vi "Test with main menus.vi"() -> ()   [LabVIEW 2019]
uses:
  Menu From Cluster.lvlib
panel:
  out "Item":string
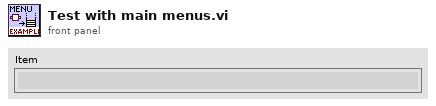
[diagram p1: front panel]
types:
  T1 = cluster{"Sub Enum":enum16{"Item1", "Item2", "Item3"}, "Sub Boolean":bool, "Subsubcluster":cluster{"Sub Enum":enum16{"Item1", "Item2", "Item3"}, "Sub Boolean":bool}}
  T2 = cluster{"An Enum":enum16{"Item1", "Item2", "Item3"}, "A Boolean":bool, "Another boolean":bool}
  T3 = cluster{"Options Menu":cluster{"An Enum":enum16{"Item1", "Item2", "Item3"}, "A Boolean":bool, "Another boolean":bool}}
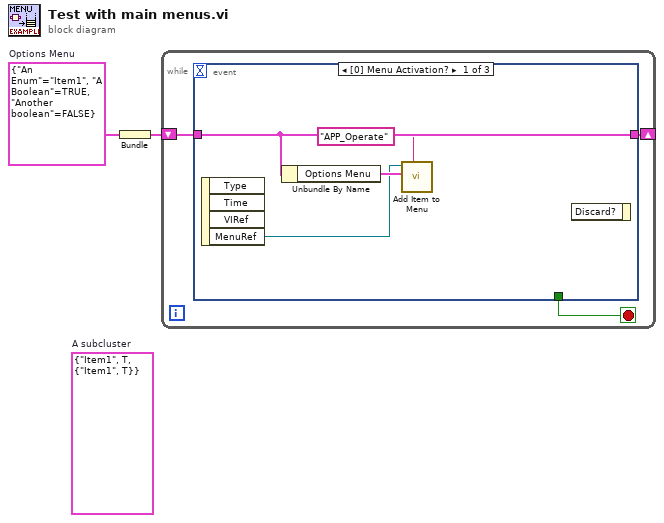
[diagram p0: block diagram]
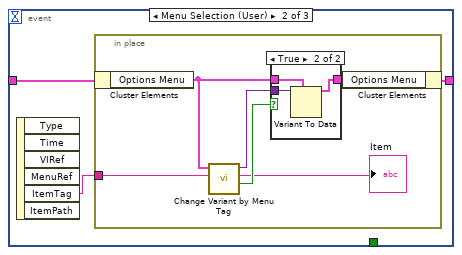
[diagram p2: hidden frame]
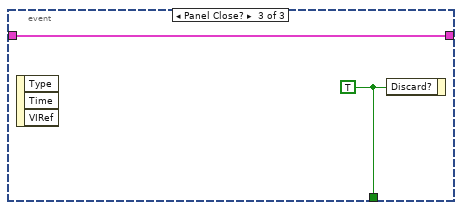
[diagram p4: hidden frame]
diagram:
  (unwired) T1 {"Sub Enum"=enum."Item1", "Sub Boolean"=TRUE, "Subsubcluster"={"Sub Enum"=enum."Item1", "Sub Boolean"=TRUE}}  # A subcluster
  w1 = T2 {"An Enum"=enum."Item1", "A Boolean"=TRUE, "Another boolean"=FALSE}  # Options Menu
  n1 = Bundle("Options Menu"=w1) -> (w2:T3)  [unwired: 1 in]
  n2 = while {
    shift-right: [w4] -> _
    shift-left: w2 -> [w5]
    stop <- w3 stop-if-true
    n3 = event shown="[0] Menu Activation?" {
      selector: _ -> [_ _ _]
      dyn-events: _ -> [_ _ _]
      timeout: _ -> [_ _ _]
      tunnel: w5 -> [w9 w12 w24]
      tunnel: [w9 w11 w24] -> w4
      tunnel: [_ _ w23] -> w3
      event Menu Activation? {
        n4 = event-data() -> ("MenuRef"=w7:refnum<k9>)  [unwired: 1 in, 3 out]
        n5 = Unbundle By Name(w9) -> ("Options Menu"=w8:T2)
        n6 = call "Add Item to Menu.vi"("menu tag"="APP_Operate", "Item(s) to Add"=w8, "menu reference"=w7) -> ()  [unwired: 6 in, 3 out]
        n7 = event-data() -> ()  [unwired: 2 in, 1 out]
      }
      event Menu Selection (User) {
        n8 = event-data() -> ("ItemTag"=w10:string)  [unwired: 1 in, 5 out]
        n9 = in-place {
          in-place-border: w10 -> [w14]
          n10 = in-place-cluster #1(w12) -> ("Options Menu"=w17:T2)
          n11 = call "Change Variant by Menu Tag.vi"("tag"=w14, "Cluster"=w17) -> ("Cluster Changed"=w15:bool, "Item"=→"Item":string, "VCluster out"=w16:variant)  [unwired: 6 in, 1 out]
          n12 = case shown="True" w15 {
            tunnel: w16 -> [_ w22]
            tunnel: [w19 w21] -> w18
            tunnel: w17 -> [w19 w20]
            frame False {
            }
            frame True {
              n13 = Variant To Data(type=w20, Variant=w22) -> (data=w21:T2)  [unwired: 1 in, 1 out]
            }
          }
          n14 = in-place-cluster #1("Options Menu"=w18) -> (w11:T3)
        }
      }
      event Panel Close? {
        w23 = TRUE
        n15 = event-data() -> ()  [unwired: 1 in, 3 out]
        n16 = event-data("Discard?"=w23) -> ()  [unwired: 1 in, 1 out]
      }
    }
  }
